vi "destroy.vi"(8 "error in":errorcluster, 11 "Nominal Client":refnum<class "Nominal Client.lvclass">) -> (0 "error out":errorcluster)   [LabVIEW 2020, in "Nominal Client.lvclass"]
uses:
  Nominal Client.lvclass
  Nominal Client.lvclass/Nominal Client.ctl
  submodules/reqwest-labview/lv-src/reqwest/reqwest.lvclass
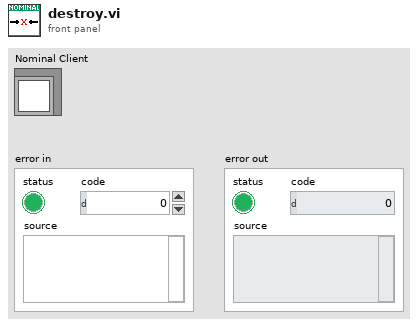
[diagram p1: front panel]
types:
  T1 = typedef "Nominal Client.lvclass/private_data.ctl" = cluster{"API Token":string, "workspace":refnum<class "workspace.lvclass">, "Available Workspaces":refnum<class "workspace.lvclass">[], "reqwest":refnum<class "reqwest.lvclass">}
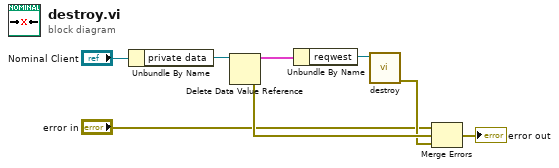
[diagram p0: block diagram]
diagram:
  n1 = Unbundle By Name("Nominal Client") -> ("private data"=w7:refnum<data-value>)
  n2 = Delete Data Value Reference(data value reference=w7) -> (data value=w6:T1, error out=w5:errorcluster)  [unwired: 1 in]
  n3 = Unbundle By Name(w6) -> ("reqwest"=w1:refnum<class "reqwest.lvclass">)
  n4 = call "destroy.vi"("reqwest"=w1) -> ("error out"=w4:errorcluster)  [unwired: 10 in]
  n5 = Merge Errors("error in", w5, w4) -> (→"error out":errorcluster)
